vi "Area of Triangle.vi"() -> ()   [LabVIEW 2022 SP3]
panel:
  out "Area of Triangle":dbl
  out "Validity of Triangle":bool
  in  "Side C":dbl=10.0
  in  "Side B":dbl=8.0
  in  "Side A":dbl=6.0
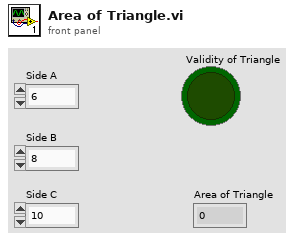
[diagram p1: front panel]
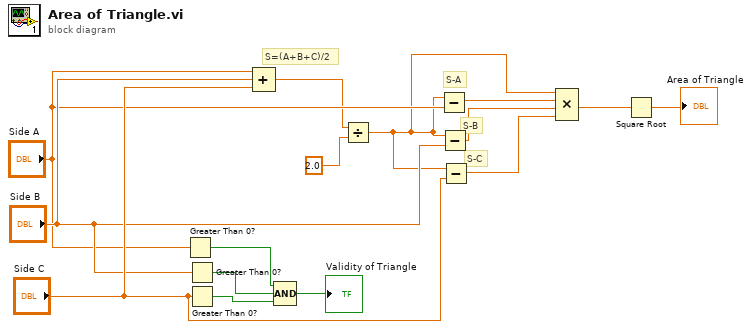
[diagram p0: block diagram]
diagram:
  # "S-C"
  # "S-B"
  # "S-A"
  # "S=(A+B+C)/2"
  n1 = Greater Than 0?(x="Side A") -> (x > 0?=w15:bool)
  n2 = Greater Than 0?(x="Side B") -> (x > 0?=w14:bool)
  n3 = Greater Than 0?(x="Side C") -> (x > 0?=w13:bool)
  n4 = Compound Arithmetic op=ADD("Side A", "Side B", "Side C") -> (w2:dbl)
  n5 = Compound Arithmetic op=AND(w15, w14, w13) -> (→"Validity of Triangle":bool)
  n6 = Divide(x=w2, y=2.0) -> (x/y=w1:dbl)
  n7 = Subtract(x=w1, y="Side A") -> (x-y=w8:dbl)
  n8 = Subtract(x=w1, y="Side B") -> (x-y=w7:dbl)
  n9 = Subtract(x=w1, y="Side C") -> (x-y=w6:dbl)
  n10 = Compound Arithmetic op=MULTIPLY(w1, w8, w7, w6) -> (w5:dbl)
  n11 = Square Root(x=w5) -> (sqrt(x)=→"Area of Triangle":dbl)
